vi "UHR-Fleezers Control (host) -TL - oscillation.vi"(0 "Tab Control":T5(tab)) -> ()   [LabVIEW 2013] (continued)
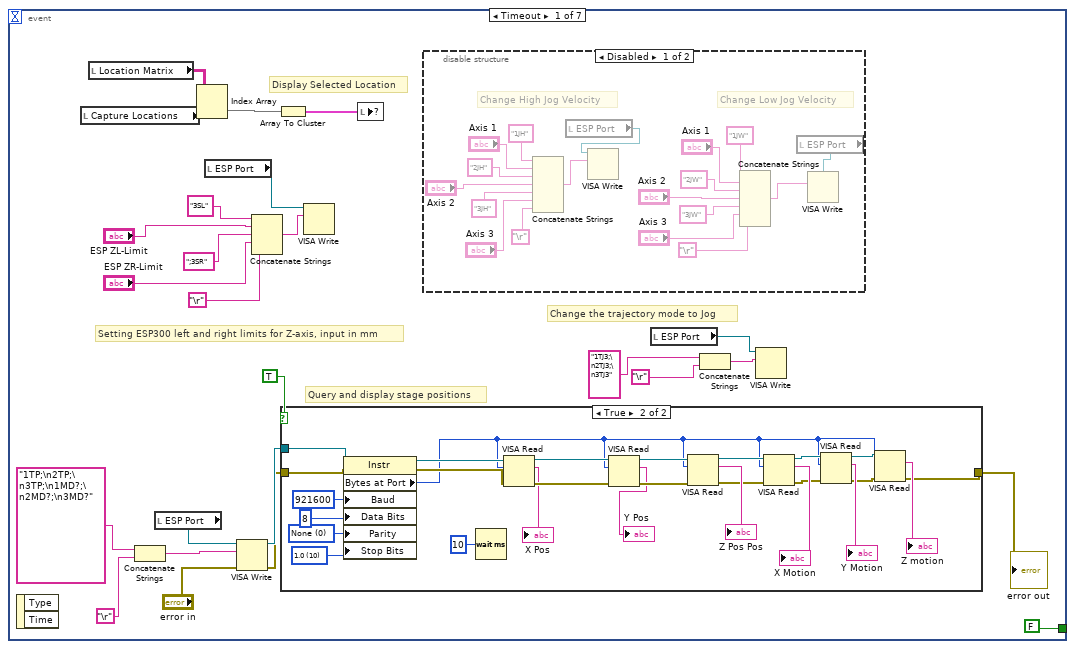
[diagram p3: hidden frame]
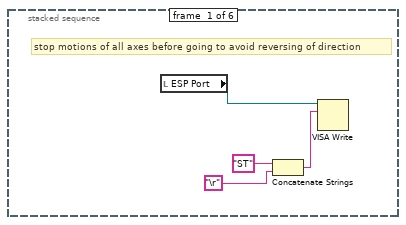
[diagram p6: hidden frame]
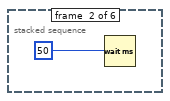
[diagram p7: hidden frame]
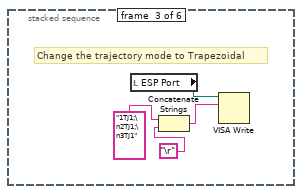
[diagram p8: hidden frame]
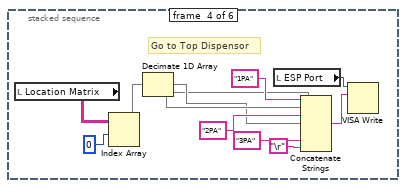
[diagram p9: hidden frame]
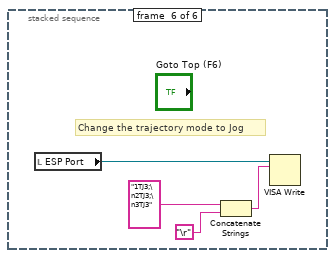
[diagram p10: hidden frame]
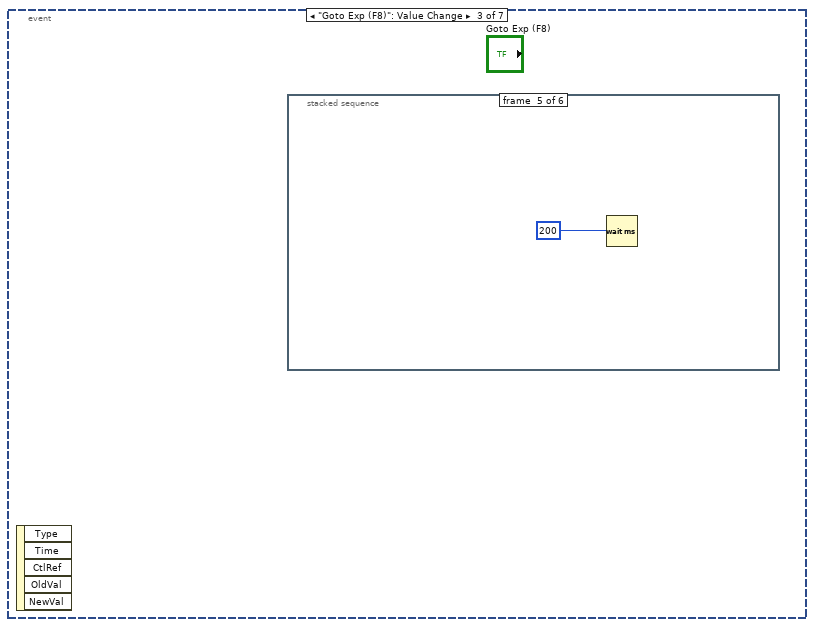
[diagram p11: hidden frame]
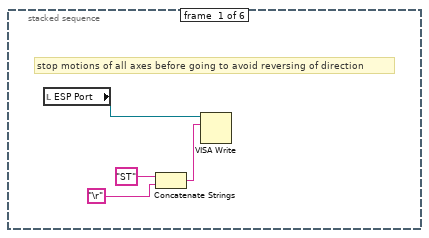
[diagram p12: hidden frame]
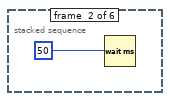
[diagram p13: hidden frame]
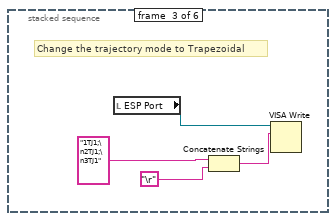
[diagram p14: hidden frame]
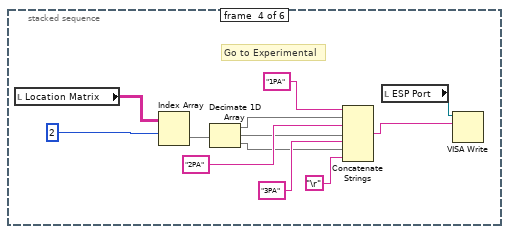
[diagram p15: hidden frame]
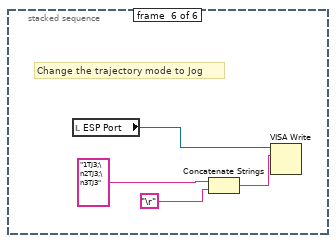
[diagram p16: hidden frame]
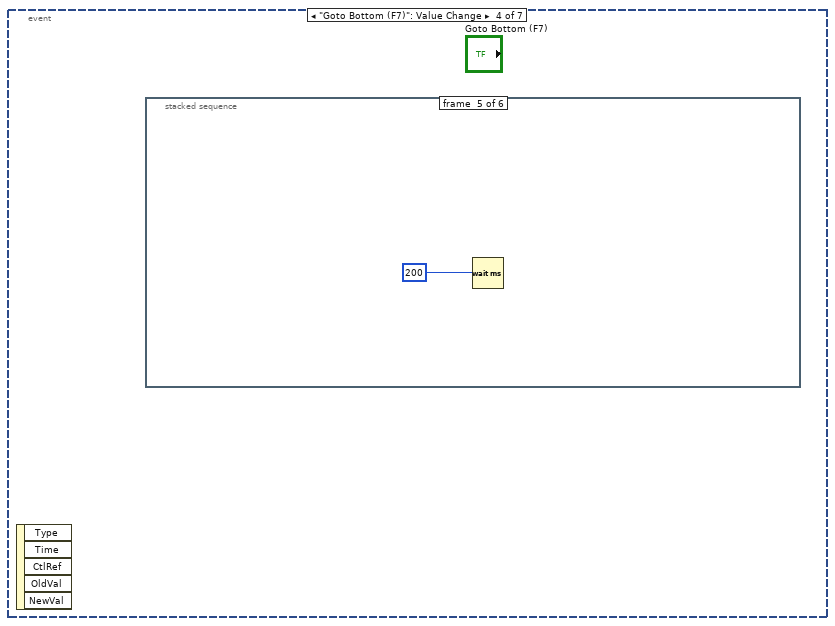
[diagram p17: hidden frame]
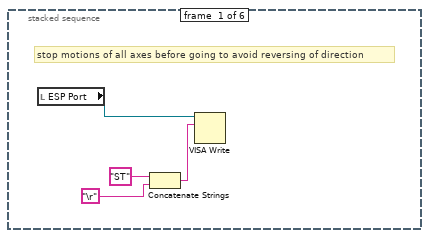
[diagram p18: hidden frame]
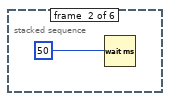
[diagram p19: hidden frame]
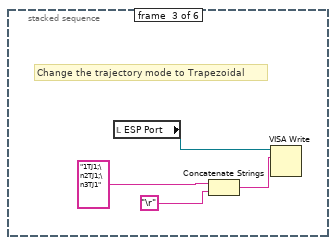
[diagram p20: hidden frame]
            n1984 = local write "Save index"(w3239) -> ()
            n1985 = Array Size(array=w3250) -> (size(s)=w3251:i32)
            n1986 = Open/Create/Replace File(file path (use dialog)=w3226, operation (0:open)=T23."create", access (0:read/write)=enum16{"read/write", "read-only", "write-only"}."write-only") -> (refnum out=w3264:refnum<file>)  [unwired: 1 in, 4 out]
            n1987 = local write "Saving..."(TRUE ("Saving...")) -> ()
            n1988 = To Double Precision Float(number=w3251) -> (double precision float=w3249:dbl)
            n1989 = String Length(string="Comment (data description)") -> (length=w3247:i32)
            n1990 = To Double Precision Float(number=w3247) -> (double precision float=w3246:dbl)
            n1991 = Deny Access(7:w3264) -> (3:w3263:refnum<file>)  [unwired: 1 in, 2 out]
            n1992 = Build Array (concatenate)(w3249, w3250, w3246) -> (w3248:dbl[])
            n1993 = case "If fluorescence data to be saved" shown="True" w3237 {
              tunnel: w3226 -> [_ w3316]
              tunnel: [refnum<k0> refnum w3296] -> w3238
              frame False {
              }
              frame True {
                w3295 = 0.0
                n1994 = local read "APD Integration Time (s)"() -> (w3301:dbl)
                n1995 = local read "N APD Samp/step"() -> (w3294:dbl)
                n1996 = Path To String(path=w3316) -> (string=w3315:string)
                n1997 = String Length(string=w3315) -> (length=w3314:i32)
                n1998 = Subtract(x=w3314, y=4) -> (x-y=w3312:i32)
                n1999 = String Subset(string=w3315, length (rest)=w3312) -> (substring=w3311:string)  [unwired: 1 out]
                n2000 = Build Array(w3301, w3294, w3295, w3295, w3295, w3295, w3295, w3295) -> (w3298:dbl[])
                n2001 = Concatenate Strings(w3311, "_fl.dat" ("string")) -> (w3309:string)
                n2002 = Array Size(array=w3298) -> (size(s)=w3300:i32)
                n2003 = String To Path(string=w3309) -> (path=w3305:path)
                n2004 = Open/Create/Replace File(file path (use dialog)=w3305, operation (0:open)=T23."create", access (0:read/write)=enum16{"read/write", "read-only", "write-only"}."write-only") -> (refnum out=w3306:refnum<file>)  [unwired: 1 in, 4 out]
                n2005 = Deny Access(7:w3306) -> (3:w3302:refnum<file>)  [unwired: 1 in, 2 out]
                n2006 = To Double Precision Float(number=w3300) -> (double precision float=w3299:dbl)
                n2007 = Build Array (concatenate)(w3299, w3298) -> (w3297:dbl[])
                n2008 = Write to Binary File(file (use dialog)=w3302, data=w3297, 5:FALSE ("prepend array or string size? (T)"), 9:T29."big-endian, network order" ("byte order (0:big-endian, network order)")) -> (refnum out=w3296:refnum<file>)  [unwired: 1 in, 3 out]
              }
            }
            n2009 = case shown="True" w3224 {
              tunnel: w3226 -> [_ w3278]
              tunnel: [refnum<k0> refnum w3277] -> w3225
              frame False {
              }
              frame True {
                w3273 = 0.0 ("element")
                n2010 = Path To String(path=w3278) -> (string=w3292:string)
                n2011 = Build Array(w3273, w3273, w3273, w3273, w3273, w3273, w3273, w3273) -> (w3274:dbl[])
                n2012 = String Length(string=w3292) -> (length=w3291:i32)
                n2013 = Subtract(x=w3291, y=4) -> (x-y=w3289:i32)
                n2014 = Array Size(array=w3274) -> (size(s)=w3276:i32)
                n2015 = String Subset(string=w3292, length (rest)=w3289) -> (substring=w3288:string)  [unwired: 1 out]
                n2016 = To Double Precision Float(number=w3276) -> (double precision float=w3275:dbl)
                n2017 = Concatenate Strings(w3288, "_pos.dat" ("string")) -> (w3286:string)
                n2018 = Build Array (concatenate)(w3275, w3274) -> (w3272:dbl[])
                n2019 = String To Path(string=w3286) -> (path=w3282:path)
                n2020 = Open/Create/Replace File(file path (use dialog)=w3282, operation (0:open)=T23."create", access (0:read/write)=enum16{"read/write", "read-only", "write-only"}."write-only") -> (refnum out=w3283:refnum<file>)  [unwired: 1 in, 4 out]
                n2021 = Deny Access(7:w3283) -> (3:w3279:refnum<file>)  [unwired: 1 in, 2 out]
                n2022 = Write to Binary File(file (use dialog)=w3279, data=w3272, 5:FALSE ("prepend array or string size? (T)"), 9:T29."big-endian, network order" ("byte order (0:big-endian, network order)")) -> (refnum out=w3277:refnum<file>)  [unwired: 1 in, 3 out]
              }
            }
            n2023 = Write to Binary File(file (use dialog)=w3263, data=w3248, 5:w3244, 9:w3242) -> (refnum out=w3245:refnum<file>)  [unwired: 1 in, 3 out]
            n2024 = Write to Binary File(file (use dialog)=w3245, data="Comment (data description)", 5:w3244, 9:w3242) -> (refnum out=w3241:refnum<file>)  [unwired: 1 in, 3 out]
          }
        }
        n2025 = feedback-in #19(w3184) -> ()
        n2026 = feedback-in #20(w3211) -> ()
        n2027 = feedback-in #21(w3183) -> ()
        n2028 = feedback-in #22(w3194) -> ()
        n2029 = feedback-in #23(w3197) -> ()
        n2030 = feedback-in #24(w3210) -> ()
        n2031 = feedback-in #25(w3200) -> ()
      }
      frame #1 {
        n2032 = local read "Saving..."() -> (w3441:bool)
        n2033 = case shown="True" w3441 {
          tunnel: w3445 -> [_ w3455]
          tunnel: w3444 -> [_ w3469]
          tunnel: w3443 -> [_ w3465]
          tunnel: w3442 -> [_ w3464]
          tunnel: w3440 -> [_ w3463]
          tunnel: w3439 -> [_ w3458]
          tunnel: w3438 -> [_ w3457]
          tunnel: w3437 -> [_ w3456]
          tunnel: w3436 -> [_ w3454]
          tunnel: w3435 -> [_ w3452]
          tunnel: w3434 -> [_ w3451]
          tunnel: w3433 -> [_ w3450]
          tunnel: w3432 -> [_ w3449]
          tunnel: w3431 -> [_ w3448]
          tunnel: w3430 -> [_ w3447]
          tunnel: w3429 -> [_ w3446]
          frame False {
          }
          frame True {
            n2034 = Multiply(x=w3455, y=w3454) -> (x*y=→"Time (s)":dbl)
            n2035 = Less Or Equal?(x=w3455, y=w3463) -> (x <= y?=w3467:bool)
            n2036 = Or(x="Stop Saving", y="Abort save 2") -> (x .or. y?=w3459:bool)
            n2037 = Not(x=w3459) -> (.not. x?=w3468:bool)
            n2038 = And(x=w3467, y=w3468) -> (x .and. y?=w3466:bool)
            n2039 = case shown="True" w3466 {
              tunnel: w3469 -> [w3476 w3544]
              tunnel: [0.0 w3547] -> w3462
              tunnel: w3455 -> [_ w3545]
              tunnel: w3463 -> [_ w3546]
              tunnel: w3465 -> [_ w3541]
              tunnel: w3464 -> [_ _]
              tunnel: w3458 -> [w3474 w3534]
              tunnel: w3457 -> [w3473 w3535]
              tunnel: w3456 -> [_ w3533]
              tunnel: w3452 -> [_ w3532]
              tunnel: w3451 -> [_ w3486]
              tunnel: w3450 -> [_ w3525]
              tunnel: w3449 -> [_ w3503]
              tunnel: w3448 -> [w3471 w3484]
              tunnel: w3447 -> [w3472 w3483]
              tunnel: w3446 -> [_ w3480]
              frame False {
                w3470 = FALSE
                n2040 = Close File(refnum=w3476) -> ()  [unwired: 1 in, 2 out]
                n2041 = case shown="True" w3473 {
                  tunnel: w3474 -> [_ w3478]
                  frame False {
                  }
                  frame True {
                    n2042 = Close File(refnum=w3478) -> ()  [unwired: 1 in, 2 out]
                  }
                }
                n2043 = case shown="True" w3471 {
                  tunnel: w3472 -> [_ w3477]
                  frame False {
                  }
                  frame True {
                    n2044 = Close File(refnum=w3477) -> ()  [unwired: 1 in, 2 out]
                  }
                }
                n2045 = local write "Calibrating Trap..."(w3470) -> ()
                n2046 = call <vilib>:"Beep.vi"() -> ()  [unwired: 3 in, 9 out]
                n2047 = local write "Stop Saving"(w3470) -> ()
                n2048 = property on="Raster Scanning..." class="Bool (strict)"("Val(Sgnl)"=w3470) -> ()  [unwired: 2 in, 2 out]
                "Saving..." <- w3470
              }
              frame True {
                n2049 = local read "Calibrating Trap..."() -> (w3536:bool)
                n2050 = case "Write fl. data" shown="True" w3535 {
                  tunnel: w3534 -> [_ w3570]
                  tunnel: w3533 -> [_ w3569]
                  frame False {
                  }
                  frame True {
                    n2051 = Write to Binary File(file (use dialog)=w3570, data=w3569, 5:FALSE ("prepend array or string size? (T)"), 9:T29."big-endian, network order" ("byte order (0:big-endian, network order)")) -> ()  [unwired: 1 in, 4 out]
                  }
                }
                n2052 = Greater?(x="Save ave N", y=1.0) -> (0:w3539:bool)
                n2053 = Not(x=w3536) -> (.not. x?=w3538:bool)
                n2054 = And(x=w3538, y=w3539) -> (x .and. y?=w3481:bool)
                n2055 = case shown="True" w3481 {
                  tunnel: w3480 -> [w3550 w3561]
                  tunnel: [w3550 w3553] -> w3479
                  tunnel: "Save ave N" -> [_ w3554]
                  frame False {
                  }
                  frame True {
                    w3551 = 2 ("dimension size")
                    n2056 = Array Size(array=w3561) -> (size(s)=w3555:i32)
                    n2057 = Divide(x=w3555, y=w3551) -> (x/y=w3559:dbl)
                    n2058 = Reshape Array(w3561, w3559, w3551) -> (w3560:u64[][])
                    n2059 = Transpose 2D Array(2D array=w3560) -> (transposed array=w3558:u64[][])
                    n2060 = for {
                      tunnel: w3558 -> [w3563] mode=indexing
                      tunnel: [w3562] -> w3552 mode=indexing
                      tunnel: w3554 -> [w3564]
                      workers-P: _ -> [_]
                      n2061 = call "downsample 1D array - U64.vi"("Ave N"=w3564, "Array In"=w3563) -> ("Array Out"=w3562:u64[])  [unwired: 1 in]
                    }
                    n2062 = Transpose 2D Array(2D array=w3552) -> (transposed array=w3557:u64[][])
                    n2063 = Divide(x=w3555, y=w3554) -> (x/y=w3556:dbl)
                    n2064 = Reshape Array(w3557, w3556) -> (w3553:u64[])
                  }
                }
                n2065 = case shown="False" w3481 {
                  tunnel: w3541 -> [w3573 w3585]
                  tunnel: [w3573 w3577] -> w3537
                  tunnel: "Save ave N" -> [_ w3578]
                  tunnel: w3532 -> [_ w3576]
                  frame False {
                    # "don't downsample data for trap calibration"
                  }
                  frame True {
                    n2066 = Array Size(array=w3585) -> (size(s)=w3579:i32)
                    n2067 = Array Size(array=w3576) -> (size(s)=w3575:i32)
                    n2068 = Divide(x=w3579, y=w3575) -> (x/y=w3583:dbl)
                    n2069 = Reshape Array(w3585, w3583, w3575) -> (w3584:i16[][])
                    n2070 = Transpose 2D Array(2D array=w3584) -> (transposed array=w3582:i16[][])
                    n2071 = for {
                      tunnel: w3582 -> [w3588] mode=indexing
                      tunnel: [w3587] -> w3574 mode=indexing
                      tunnel: w3578 -> [w3586]
                      workers-P: _ -> [_]
                      n2072 = call "downsample 1D array - I16.vi"("Ave N"=w3586, "Array In"=w3588) -> ("Array Out"=w3587:i16[])  [unwired: 1 out]
                    }
                    n2073 = Transpose 2D Array(2D array=w3574) -> (transposed array=w3581:i16[][])
                    n2074 = Divide(x=w3579, y=w3578) -> (x/y=w3580:dbl)
                    n2075 = Reshape Array(w3581, w3580) -> (w3577:i16[])
                  }
                }
                n2076 = Index Array(array=w3503, index=1) -> (element=w3506:waveform(dbl))
                n2077 = Index Array(array=w3503, index=0) -> (element=w3508:waveform(dbl))
                n2078 = Unbundle By Name(w3506) -> ("Y"=w3510:dbl[])
                n2079 = Unbundle By Name(w3508) -> ("Y"=w3518:dbl[])
                n2080 = case "Write trap pos. data" shown="True" w3484 {
                  tunnel: w3483 -> [_ w3566]
                  tunnel: w3479 -> [_ w3565]
                  frame False {
                  }
                  frame True {
                    n2081 = Write to Binary File(file (use dialog)=w3566, data=w3565, 5:FALSE ("prepend array or string size? (T)"), 9:T29."big-endian, network order" ("byte order (0:big-endian, network order)")) -> ()  [unwired: 1 in, 4 out]
                  }
                }
                n2082 = Write to Binary File(file (use dialog)=w3544, data=w3537, 5:FALSE ("prepend array or string size? (T)"), 9:T29."big-endian, network order" ("byte order (0:big-endian, network order)")) -> ()  [unwired: 1 in, 4 out]
                n2083 = feedback #26(w3510) -> (w3512:dbl[])
                n2084 = Build Array (concatenate)(w3512, w3510) -> (w3511:dbl[])
                n2085 = Select(t=w3510, s=w3486, f=w3511) -> (s? t:f=w3496:dbl[])
                n2086 = feedback-in #26(w3496) -> ()
                n2087 = feedback #27(w3518) -> (w3531:dbl[])
                n2088 = Build Array (concatenate)(w3531, w3518) -> (w3530:dbl[])
                n2089 = Select(t=w3518, s=w3486, f=w3530) -> (s? t:f=w3505:dbl[])
                n2090 = feedback-in #27(w3505) -> ()
                n2091 = Divide(x=w3545, y=w3546) -> (x/y=w3548:dbl)
                n2092 = Multiply(x=w3548, y=100.0) -> (x*y=w3547:dbl)
                n2093 = Build Array(w3505, w3496) -> (→"Saved APD":dbl[][])
                n2094 = Array Size(array=w3505) -> (size(s)=w3523:i32)
                n2095 = Unbundle By Name(w3525) -> ("Y"=w3529:dbl[])
                n2096 = Subtract(x=w3523, y="N pts to average") -> (x-y=w3499:i32)
                n2097 = Multiply(x="N pts to average", y=u16 2) -> (x*y=w3500:u16)
                n2098 = Subtract(x=w3523, y=w3500) -> (x-y=w3498:i32)
                n2099 = feedback #28(w3529) -> (w3528:dbl[])
                n2100 = Build Array (concatenate)(w3528, w3529) -> (w3527:dbl[])
                n2101 = Select(t=w3529, s=w3486, f=w3527) -> (s? t:f=w3526:dbl[])
                "Trap Delta Graph" <- w3526
                n2102 = feedback-in #28(w3526) -> ()
                n2103 = Array Subset(array=w3505, index=w3499, length="N pts to average") -> (w3522:dbl[])
                n2104 = Array Subset(array=w3505, index=w3498, length="N pts to average") -> (w3521:dbl[])
                n2105 = Array Subset(array=w3496, index=w3499, length="N pts to average") -> (w3502:dbl[])
                n2106 = Array Subset(array=w3496, index=w3498, length="N pts to average") -> (w3501:dbl[])
                n2107 = call-poly <vilib>:"Mean.vi"("X"=w3522) -> ("mean"=w3520:dbl)  [unwired: 1 out]
                n2108 = call-poly <vilib>:"Mean.vi"("X"=w3502) -> ("mean"=w3495:dbl)  [unwired: 1 out]
                n2109 = call-poly <vilib>:"Mean.vi"("X"=w3521) -> ("mean"=w3519:dbl)  [unwired: 1 out]
                n2110 = call-poly <vilib>:"Mean.vi"("X"=w3501) -> ("mean"=w3494:dbl)  [unwired: 1 out]
                n2111 = Subtract(x=w3495, y=w3494) -> (x-y=w3485:dbl)
                "Delta Fl. 2" <- w3485
                n2112 = Subtract(x=w3520, y=w3519) -> (x-y=w3517:dbl)
                "Delta Fl. 1" <- w3517
                n2113 = Initialize Array(w3517, 1 ("dimension size")) -> (w3514:dbl[])
                n2114 = Initialize Array(w3485, 1 ("dimension size")) -> (w3491:dbl[])
                n2115 = feedback #29(w3514) -> (w3515:dbl[])
                n2116 = Build Array (concatenate)(w3515, w3514) -> (w3513:dbl[])
                n2117 = feedback #30(w3491) -> (w3492:dbl[])
                n2118 = Build Array (concatenate)(w3492, w3491) -> (w3490:dbl[])
                n2119 = Select(t=w3514, s=w3486, f=w3513) -> (s? t:f=w3489:dbl[])
                n2120 = feedback-in #29(w3489) -> ()
                n2121 = Select(t=w3491, s=w3486, f=w3490) -> (s? t:f=w3488:dbl[])
                n2122 = feedback-in #30(w3488) -> ()
                n2123 = Build Array(w3489, w3488) -> (→"Save APD Deriv":dbl[][])
              }
            }
            "Progress" <- w3462
            "Progress 2" <- w3462
          }
        }
      }
    }
    n2124 = Bundle By Name(cluster=w2208, "Green FB Ch 0"=w2207, "Green FB Ch 1"=w2206) -> (w2186:T48)
    "Green FB Signals (V)" <- w2186
    n2125 = Unbundle By Name(w2186) -> ("Green FB Ch 2"=→"Green FB Plot":dbl)
    n2126 = local read "wait to reset values"() -> (w2276:bool)
    n2127 = Not(x=w2273) -> (.not. x?=w2277:bool)
    n2128 = And(x=w2277, y=w2276) -> (x .and. y?=w2278:bool)
    n2129 = case "Part of MCL raster scanning: returns to initial positions after scan done" shown="False" w2278 {
      tunnel: w2281 -> [w3014 w3021]
      tunnel: [w3014 w3020] -> w2280
      tunnel: w2275 -> [w3013 w3019]
      tunnel: [w3013 w3018] -> w2274
      frame False {
      }
      frame True {
        w3029 = 10.0 ("y")
        w3028 = 32767.0 ("y")
        # "to return scan values\nafter a synchronous \nAOM scan"
        n2130 = local read "AO2"() -> (w3022:dbl)
        n2131 = local read "AO1"() -> (w3023:dbl)
        n2132 = local write "wait to reset values"(FALSE ("wait to reset values")) -> ()
        n2133 = Multiply(x=w3023, y=w3028) -> (x*y=w3025:dbl)
        n2134 = Multiply(x=w3022, y=w3028) -> (x*y=w3027:dbl)
        n2135 = Divide(x=w3025, y=w3029) -> (x/y=w3024:dbl)
        n2136 = Divide(x=w3027, y=w3029) -> (x/y=w3026:dbl)
        n2137 = To Word Integer(number=w3024) -> (16bit integer=w3030:i16)
        n2138 = To Word Integer(number=w3026) -> (16bit integer=w3031:i16)
        n2139 = local read "Total Counts (ticks)"() -> (w3015:u32)
        n2140 = xnode "Read/Write Control"("FPGA VI Reference In"=w3021, "error in"=w3019, "AO1"=w3030, "AO2"=w3031, "MCL count"=w3015) -> ("FPGA VI Reference Out"=w3020:T19, "error out"=w3018:errorcluster)
        n2141 = local read "Scan Range (V)\n(of steps)"() -> (w3016:dbl)
        n2142 = property on="Scan Range (V)\n(of steps)" class="DigNum (strict)"("Val(Sgnl)"=w3016) -> ()  [unwired: 2 in, 2 out]
      }
    }
    n2143 = node-c288() -> ()  [unwired: 2 out]
  }
  n2144 = node-c288(3 ("Processor")) -> (w77:T24)  [unwired: 3 out]
  n2145 = timed-loop "Oscillate AOD (debugging)" {
    tunnel: w2 -> [w3590]
    tunnel: [w3589] -> w40
    timing: w77 -> [_]
    timing-out: [_] -> w76
    stop <- w3589 stop-if-true
    n2146 = node-c288() -> ()  [unwired: 2 out]
    n2147 = event shown="[0] \"Oscillate Traps\", \"Fish for Tether\": Value Change" {
      selector: _ -> [_ _ _]
      dyn-events: _ -> [_ _ _]
      timeout: _ -> [_ _ _]
      tunnel: w3590 -> [w3597 _ _]
      tunnel: [FALSE ("Stop All") _ w3869] -> w3589
      event "Oscillate Traps", "Fish for Tether": Value Change {
        n2148 = event-data() -> ()  [unwired: 6 out]
        n2149 = local read "Oscillate Traps"() -> (w3596:bool)
        n2150 = Or(x=w3596, y="Fish for Tether") -> (x .or. y?=w3594:bool)
        n2151 = case shown="True" w3594 {
          tunnel: w3597 -> [_ w3600]
          tunnel: "Fish for Tether" -> [_ w3599]
          frame False {
          }
          frame True {
            n2152 = case shown="True" w3599 {
              frame False {
              }
              frame True {
                n2153 = local write "Scan axis (osc)"(TRUE) -> ()
                n2154 = local write "Tether"(FALSE ("Tether")) -> ()
              }
            }
            n2155 = node-c288("Time Step (ms)") -> (w3602:T24)  [unwired: 3 out]
            n2156 = timed-loop "Oscillate AOD" {
              timing: w3602 -> [_]
              timing-out: [_] -> w3601
              tunnel: w3600 -> [w3612]
              tunnel: w3599 -> [w3611]
              i -> [w3614]
              stop <- w3610 stop-if-true
              n2157 = node-c288() -> (w3613:i64)  [unwired: 1 out]
              n2158 = flat-sequence {
                tunnel: w3614 -> [w3643]
                tunnel: w3613 -> [w3642]
                tunnel: w3612 -> [w3628]
                tunnel: w3611 -> [w3630]
                tunnel: [w3630] -> w3609
                tunnel: [w3629] -> w3608
                tunnel: [w3627] -> w3607
                tunnel: [w3624] -> w3605
                tunnel: w3609 -> [w3680]
                tunnel: w3608 -> [w3678]
                tunnel: w3607 -> [w3677]
                tunnel: [w3676] -> w3606
                tunnel: w3605 -> [w3675]
                tunnel: [w3744] -> w3610
                tunnel: w3606 -> [w3742]
                frame #0 {
                  # "Also note that the 1 ms lower limit per iteration of all LabView loops\nis the reason why the power spectrum shows higher harmonics\nwhen performing a forced oscillation-based calibration procedure.\nOne solution to this would be to implement the osciallation using\nthe FPGA, or to account for the harmonics in the analysis. The forced\noscillation needs to discretized on timescales that won't affect\nthe power spectrum (i.e., > 66 kHz detection bandwidth; < 15 µs)."
                  # "Note: Trap Oscillation was originally written\nfor Trap 2!!!  This was modified to oscillation\nboth traps for board 1 (x-axis), but not changed\nfor board 2 (y-axis), since we only implement\nx-axis control at the moment (TL, 1/1/15)"
                  n2159 = Divide(x=w3642, y=i64 1000) -> (x/y=w3637:dbl)
                  n2160 = Multiply(x=w3637, y=w3643) -> (x*y=w3639:dbl)
                  n2161 = Multiply(x="Osc. freq. (Hz)", y=6.283185307179586) -> (x*y=w3640:dbl)
                  n2162 = Multiply(x=w3640, y=w3639) -> (x*y=w3626:dbl)
                  n2163 = local read "BD 1 Frequency 1 (MHz)"() -> (w3616:dbl)
                  n2164 = local read "BD 1 Frequency 2 (MHz)"() -> (w3623:dbl)
                  n2165 = case shown="False" w3630 {
                    tunnel: w3626 -> [w3649 w3657]
                    tunnel: w3623 -> [_ w3667]
                    tunnel: [w3644 w3651] -> w3618
                    tunnel: [FALSE w3660] -> w3627
                    tunnel: [0.0 w3653] -> w3624
                    tunnel: w3616 -> [_ w3652]
                    tunnel: [w3644 0.0 ("y")] -> w3615
                    frame False {
                      n2166 = Sine(x=w3649) -> (sin(x)=w3647:dbl)
                      n2167 = Multiply(x=w3647, y="Osc. amp. (MHz)") -> (x*y=w3644:dbl)
                    }
                    frame True {
                      n2168 = Cosine(x=w3657) -> (cos(x)=w3670:dbl)
                      n2169 = Subtract(x=w3667, y=w3652) -> (x-y=w3666:dbl)
                      n2170 = Decrement(x=w3670) -> (x-1=w3669:dbl)
                      n2171 = Subtract(x=w3666, y="Closest Delta (MHz)") -> (x-y=w3663:dbl)
                      n2172 = Divide(x=w3669, y=2.0) -> (x/y=w3664:dbl)
                      n2173 = Multiply(x=w3664, y=w3663) -> (x*y=w3651:dbl)
                      n2174 = local read "Vec Mean of T1 T2"() -> (w3659:dbl[])
                      n2175 = Greater?(x=w3659, y="Stop F (pN)") -> (0:w3661:bool[])
                      n2176 = Or Array Elements(Boolean array=w3661) -> (logical OR=w3660:bool)
                      n2177 = Divide(x=w3657, y=6.283185307179586) -> (x/y=w3656:dbl)
                      n2178 = Round Toward +Infinity(x=w3656) -> (ceil(x): smallest int >= x=w3653:dbl)
                      "Attempts" <- w3653
                      n2179 = Greater?(x=w3653, y="Attempt Limit") -> (0:w3655:bool)
                      n2180 = case shown="True" w3655 {
                        frame False {
                        }
                        frame True {
                          n2181 = local write "Fish for Tether"(FALSE ("Fish for Tether")) -> ()
                          n2182 = call <vilib>:"Beep.vi"() -> ()  [unwired: 3 in, 9 out]
                          n2183 = local read "Messages"() -> (w3672:string)
                          n2184 = call "Update messages.vi"("Message to add"="Tether fishing timeout." ("Messages"), "Old message string"=w3672) -> ("New message string"=→"Messages":string)
                        }
                      }
                    }
                  }
                  n2185 = Add(x=w3615, y=w3616) -> (x+y=w3620:dbl)
                  n2186 = Select(t=w3620, s="Scan axis (osc)", f=w3616) -> (s? t:f=w3617:dbl)
                  n2187 = local read "Y RF Frequency Limits (MHz)"() -> (w3631:T16)
                  n2188 = local read "X RF Frequency Limits (MHz)"() -> (w3632:T16)
                  n2189 = local read "BD 2 Frequency 2 (MHz)"() -> (w3622:dbl)
                  n2190 = Select(t=w3623, s="Scan axis (osc)", f=w3622) -> (s? t:f=w3633:dbl)
                  n2191 = Add(x=w3618, y=w3633) -> (x+y=w3629:dbl)
                  n2192 = Select(t=w3629, s="Scan axis (osc)", f=w3623) -> (s? t:f=w3621:dbl)
                  n2193 = Select(t=w3622, s="Scan axis (osc)", f=w3629) -> (s? t:f=w3634:dbl)
                  n2194 = local read "BD 2 Frequency 3 (MHz)"() -> (w3635:dbl)
                  n2195 = local read "BD 1 Frequency 3 (MHz)"() -> (w3636:dbl)
                  n2196 = call "set RF board frequency - interlace.vi"("Board 2 Frequency Limits"=w3631, "Board 1 Frequency Limits"=w3632, "FPGA VI Reference In"=w3628, "Board 2 Frequency 3 (MHz)"=w3635, "Board 1 Frequency 3 (MHz)"=w3636, "Board 2 Frequency 2 (MHz)"=w3622, "Board 2 Frequency 1 (MHz)"=w3634, "Board 1 Frequency 2 (MHz)"=w3621, "Board 1 Frequency 1  (MHz)"=w3617) -> ()  [unwired: 1 in, 2 out]
                }
                frame #1 {
                  n2197 = And(x=w3680, y=w3677) -> (x .and. y?=w3679:bool)
                  n2198 = case "Only if were fishing and now formed tether" shown="True" w3679 {
                    tunnel: w3678 -> [w3682 w3694]
                    tunnel: [w3681 w3693] -> w3676
                    tunnel: w3675 -> [_ w3689]
                    frame False {
                      n2199 = local read "Fish for Tether"() -> (w3681:bool)
                      n2200 = case shown="True" w3681 {
                        tunnel: w3682 -> [_ _]
                        frame False {
                        }
                        frame True {
                        }
                      }
                    }
                    frame True {
                      w3693 = FALSE ("Fish for Tether")
                      n2201 = call <vilib>:"Beep.vi"() -> ()  [unwired: 3 in, 9 out]
                      n2202 = Number To Decimal String(number=w3689, width (-)=i16 1) -> (decimal integer string=w3687:string)
                      n2203 = case shown="\"2\", \"3\", \"4\", \"5\", \"6\"" "Then..." {
                        selector: "Then..." -> [_ w3697]
                        tunnel: w3694 -> [w3696 _]
                        frame "1", Default {
                          # "do nothing"
                          n2204 = property on="BD 1 Frequency 1 (MHz)" class="DigNum (strict)"("Val(Sgnl)"=w3696) -> ()  [unwired: 2 in, 2 out]
                        }
                        frame "2", "3", "4", "5", "6" {
                          n2205 = flat-sequence {
                            tunnel: w3697 -> [w3699]
                            frame #0 {
                              n2206 = property on="Trap Delta (MHz)" class="DigNum (strict)"("Val(Sgnl)"="Move to Delta 1 (MHz)") -> ()  [unwired: 2 in, 2 out]
                            }
                            frame #1 {
                              n2207 = case shown="\"5\", \"6\"" w3699 {
                                selector: w3699 -> [w3702 w3712 _]
                                frame "3", "4" {
                                n2208 = flat-sequence {
                                tunnel: w3702 -> [w3703]
                                tunnel: [w3703] -> w3700
                                tunnel: [w3705] -> w3701
                                tunnel: w3700 -> [w3705]
                                tunnel: w3701 -> [w3709]
                                frame #0 {
                                n2209 = property on="Green Laser ON/Interlacing" class="Bool (strict)"("Val(Sgnl)"=TRUE ("Value (Signaling)")) -> ()  [unwired: 2 in, 2 out]
                                }
                                frame #1 {
                                n2210 = Multiply(x="Wait Before Save (s)", y=u32 1000 ("x")) -> (x*y=w3707:u32)
                                n2211 = Wait (ms)(milliseconds to wait=w3707) -> ()  [unwired: 1 out]
                                }
                                frame #2 {
                                n2212 = property on="Start Saving" class="Bool (strict)"("Value"=TRUE ("Start Saving")) -> ()  [unwired: 2 in, 2 out]
                                n2213 = case shown="Default" w3709 {
                                frame Default {
                                }
                                frame "4" {
                                n2214 = property on="Fl. Triggered..." class="Bool (strict)"("Val(Sgnl)"=TRUE ("Value (Signaling)")) -> ()  [unwired: 2 in, 2 out]
                                }
                                }
                                }
                                }
                                }
                                frame "5", "6" {
                                n2215 = stacked-sequence {
                                tunnel: w3712 -> [_ _ _ _ _ _ _ _ w3729 _ _]
                                frame #0 {
                                n2216 = Replace Array Subset(array=u32[] [0] ("Index Values"), new element="Raster Set Upon Tether", index=0) -> (w3713:u32[])
                                n2217 = property on="Saved AOD Raster Scan Parameter Sets" class="Arr (strict)"("Index Values"=w3713) -> ()  [unwired: 2 in, 2 out]
                                }
                                frame #1 {
                                n2218 = Wait (ms)(milliseconds to wait=u32 500) -> ()  [unwired: 1 out]
                                }
                                frame #2 {
                                n2219 = property on="Load parameters" class="Bool (strict)"("Val(Sgnl)"=TRUE ("Value (Signaling)")) -> ()  [unwired: 2 in, 2 out]
                                }
                                frame #3 {
                                n2220 = Wait (ms)(milliseconds to wait=u32 500) -> ()  [unwired: 1 out]
                                }
                                frame #4 {
                                n2221 = property on="Trap Raster Scan" class="Bool (strict)"("Val(Sgnl)"=TRUE ("Value (Signaling)")) -> ()  [unwired: 2 in, 2 out]
                                }
                                frame #5 {
                                n2222 = Wait (ms)(milliseconds to wait=u32 2000) -> ()  [unwired: 1 out]
                                }
                                frame #6 {
                                n2223 = while {
                                stop <- w3724 stop-if-true
                                n2224 = local read "Raster Scanning..."() -> (w3723:bool)
                                n2225 = local read "Saving..."() -> (w3726:bool)
                                n2226 = Wait (ms)(milliseconds to wait=u32 100) -> ()  [unwired: 1 out]
                                n2227 = Not(x=w3726) -> (.not. x?=w3725:bool)
                                n2228 = Not(x=w3723) -> (.not. x?=w3722:bool)
                                n2229 = And(x=w3725, y=w3722) -> (x .and. y?=w3724:bool)
                                }
                                }
                                frame #7 {
                                n2230 = property on="Trap Delta (MHz)" class="DigNum (strict)"("Val(Sgnl)"="Move to Delta 2 (MHz)") -> ()  [unwired: 2 in, 2 out]
                                }
                                frame #8 {
                                n2231 = local read "Tether"() -> (w3730:bool)
                                n2232 = case shown="True" w3730 {
                                tunnel: w3729 -> [_ w3731]
                                frame False {
                                }
                                frame True {
                                n2233 = flat-sequence {
                                tunnel: w3731 -> [w3733]
                                frame #0 {
                                n2234 = Wait (ms)(milliseconds to wait=u32 500) -> ()  [unwired: 1 out]
                                }
                                frame #1 {
                                n2235 = case shown="\"6\"" w3733 {
                                frame Default {
                                }
                                frame "6" {
                                n2236 = property on="Green Laser ON/Interlacing" class="Bool (strict)"("Val(Sgnl)"=TRUE ("Green Laser ON/Interlacing")) -> ()  [unwired: 2 in, 2 out]
                                }
                                }
                                }
                                frame #2 {
                                n2237 = Wait (ms)(milliseconds to wait=u32 500) -> ()  [unwired: 1 out]
                                }
                                frame #3 {
                                n2238 = local write "Start Saving"("Save at end (5, 6)") -> ()
                                }
                                }
                                }
                                }
                                }
                                frame #9 {
                                n2239 = local read "Bead Sep. Int. Time (s)"() -> (w3739:dbl)
                                n2240 = Multiply(x=w3739, y=1000.0) -> (x*y=w3738:dbl)
                                n2241 = Wait (ms)(milliseconds to wait=w3738) -> ()  [unwired: 1 out]
                                }
                                frame #10 {
                                n2242 = property on="Rescale on Mean" class="Bool (strict)"("Val(Sgnl)"=TRUE ("Value (Signaling)")) -> ()  [unwired: 2 in, 2 out]
                                }
                                }
                                }
                                frame "2", Default {
                                }
                              }
                            }
                          }
                        }
                      }
                      n2243 = Concatenate Strings("Formed tether in ", w3687, " attempt(s)." ("string")) -> (w3684:string)
                      n2244 = local read "Messages"() -> (w3691:string)
                      n2245 = local write "Fish for Tether"(w3693) -> ()
                      n2246 = call "Update messages.vi"("Message to add"=w3684, "Old message string"=w3691) -> ("New message string"=w3690:string)
                      n2247 = local write "Messages"(w3690) -> ()
                      n2248 = Get Date/Time In Seconds() -> (seconds since 1Jan1904=→"Time tether formed":timestamp)
                      "Tether" <- "Tether Alarm?"
                    }
                  }
                }
                frame #2 {
                  n2249 = local read "Oscillate Traps"() -> (w3743:bool)
                  n2250 = local read "Stop All"() -> (w3745:bool)
                  n2251 = Not Or(1:w3742, 2:w3743) -> (0:w3741:bool)
                  n2252 = Compound Arithmetic op=OR(w3745, w3741) -> (w3744:bool)
                }
              }
              n2253 = node-c288() -> ()  [unwired: 2 out]
            }
            n2254 = node-c288(w3601) -> ()  [unwired: 1 out]
          }
        }
      }
      event "Fl. Triggered...": Value Change {
        n2255 = event-data() -> ()  [unwired: 7 out]
        n2256 = case shown="True" "Fl. Triggered..." {
          frame False {
          }
          frame True {
            n2257 = node-c288() -> (w3757:T24)  [unwired: 4 out]
            n2258 = timed-loop {
              timing: w3757 -> [_]
              timing-out: [_] -> w3756
              tunnel: "Action" -> [w3761]
              shift-right: [w3758] -> _
              shift-left: u8 255 -> [w3760]
              stop <- w3762 stop-if-true
              n2259 = node-c288() -> ()  [unwired: 2 out]
              n2260 = flat-sequence {
                tunnel: w3761 -> [w3774]
                tunnel: w3760 -> [w3771]
                tunnel: [w3770] -> w3759
                tunnel: [w3860] -> w3762
                tunnel: w3759 -> [w3859]
                tunnel: [w3859] -> w3758
                frame #0 {
                  n2261 = local read "Delta Fl. 2"() -> (w3765:dbl)
                  n2262 = local read "Delta Fl. 1"() -> (w3766:dbl)
                  n2263 = Select(t=w3766, s="APD to Watch", f=w3765) -> (s? t:f=w3764:dbl)
                  n2264 = Multiply(x="Fl. Delta Thresh. (kHz)", y=1000.0) -> (x*y=w3773:dbl)
                  n2265 = Greater?(x=w3764, y=w3773) -> (0:w3768:bool)
                  n2266 = Or(x="Force Yank", y=w3768) -> (x .or. y?=w3769:bool)
                  n2267 = case shown="True" w3769 {
                    tunnel: w3774 -> [_ w3784]
                    tunnel: w3771 -> [w3776 w3780]
                    tunnel: [w3776 w3777] -> w3770
                    frame False {
                    }
                    frame True {
                      n2268 = flat-sequence {
                        tunnel: w3781 -> [w3790]
                        tunnel: [w3790] -> w3785
                        tunnel: w3784 -> [w3789]
                        tunnel: [w3789] -> w3783
                        tunnel: [w3788] -> w3782
                        tunnel: w3780 -> [w3787]
                        tunnel: [w3786] -> w3779
                        tunnel: w3785 -> [w3815]
                        tunnel: w3783 -> [w3814]
                        tunnel: w3782 -> [w3813]
                        tunnel: w3779 -> [w3812]
                        tunnel: [w3812] -> w3778
                        tunnel: w3778 -> [w3857]
                        tunnel: [w3857] -> w3777
                        frame #0 {
                          n2269 = call <vilib>:"Beep.vi"() -> ()  [unwired: 3 in, 9 out]
                          n2270 = local write "Waiting"(FALSE ("Waiting")) -> ()
                          n2271 = Increment(x=w3787) -> (x+1=w3786:u8)
                          n2272 = case shown="\"Yank\"" w3789 {
                            tunnel: w3786 -> [_ _ w3796]
                            frame "Image" {
                              n2273 = property on="Confocal Image" class="Bool (strict)"("Val(Sgnl)"=TRUE ("Value (Signaling)")) -> ()  [unwired: 2 in, 2 out]
                            }
                            frame "Alarm", Default {
                            }
                            frame "Yank" {
                              n2274 = flat-sequence {
                                tunnel: w3796 -> [w3799]
                                tunnel: [w3798] -> w3795
                                tunnel: ["N Array El"] -> w3794
                                tunnel: w3795 -> [w3809]
                                tunnel: w3794 -> [w3805]
                                frame #0 {
                                n2275 = Multiply(x="Yank Delay (s)", y=1000.0) -> (x*y=w3802:dbl)
                                n2276 = Quotient & Remainder(x=w3799, y="N Array El") -> (x-y*floor(x/y)=w3798:u8)  [unwired: 1 out]
                                n2277 = Wait (ms)(milliseconds to wait=w3802) -> ()  [unwired: 1 out]
                                }
                                frame #1 {
                                n2278 = Random Number (0-1)() -> (number: 0 to 1=w3806:dbl)
                                n2279 = Multiply(x=w3805, y=w3806) -> (x*y=w3804:dbl)
                                n2280 = Round Toward -Infinity(1:w3804) -> (0:w3803:dbl)
                                n2281 = Select(t=w3803, s="Random Choice", f=w3809) -> (s? t:f=w3807:dbl)
                                n2282 = Index Array(array="Yank to Delta Array (MHz)", index=w3807) -> (element=w3810:dbl)
                                n2283 = property on="Trap Delta (MHz)" class="DigNum (strict)"("Val(Sgnl)"=w3810) -> ()  [unwired: 2 in, 2 out]
                                }
                              }
                            }
                          }
                          n2284 = local read "Time (s)"() -> (w3788:dbl)
                          "Fl. High" <- TRUE ("Yanking")
                        }
                        frame #1 {
                          n2285 = node-c288() -> (w3817:T24)  [unwired: 4 out]
                          n2286 = timed-loop {
                            timing: w3817 -> [_]
                            timing-out: [_] -> w3816
                            tunnel: w3815 -> [w3833]
                            tunnel: w3814 -> [w3831]
                            tunnel: w3813 -> [w3830]
                            stop <- w3832 stop-if-true
                            n2287 = node-c288() -> ()  [unwired: 2 out]
                            n2288 = local read "Fl. Delta Thresh. (kHz)"() -> (w3825:dbl)
                            n2289 = local read "Fl. Triggered..."() -> (w3834:bool)
                            n2290 = local read "Delta Fl. 1"() -> (w3821:dbl)
                            n2291 = local read "Delta Fl. 2"() -> (w3819:dbl)
                            n2292 = local read "Stop All"() -> (w3828:bool)
                            n2293 = local read "APD to Watch"() -> (w3820:bool)
                            n2294 = Select(t=w3821, s=w3820, f=w3819) -> (s? t:f=w3818:dbl)
                            n2295 = Not(x=w3834) -> (.not. x?=w3829:bool)
                            n2296 = Multiply(x=w3825, y=1000.0) -> (x*y=w3824:dbl)
                            n2297 = Negate(x=w3824) -> (-x=w3823:dbl)
                            n2298 = Less?(x=w3818, y=w3823) -> (x < y?=w3827:bool)
                            n2299 = Compound Arithmetic op=OR(w3827, w3828, w3829, "Force Reset") -> (w3832:bool)
                            n2300 = case shown="True" w3832 {
                              tunnel: w3833 -> [_ w3845]
                              tunnel: w3831 -> [_ w3844]
                              tunnel: w3830 -> [_ w3842]
                              frame False {
                              }
                              frame True {
                                n2301 = case shown="\"Yank\"" w3844 {
                                tunnel: w3845 -> [_ w3846]
                                frame "Image", Default {
                                }
                                frame "Yank" {
                                n2302 = flat-sequence {
                                tunnel: [w3851] -> w3847
                                tunnel: w3846 -> [w3851]
                                tunnel: w3847 -> [w3852]
                                frame #0 {
                                n2303 = local read "Yank Delay (s)"() -> (w3850:dbl)
                                n2304 = Multiply(x=w3850, y=1000.0) -> (x*y=w3848:dbl)
                                n2305 = Wait (ms)(milliseconds to wait=w3848) -> ()  [unwired: 1 out]
                                }
                                frame #1 {
                                n2306 = property on="Trap Delta (MHz)" class="DigNum (strict)"("Val(Sgnl)"=w3852) -> ()  [unwired: 2 in, 2 out]
                                }
                                }
                                }
                                }
                                n2307 = local read "Time (s)"() -> (w3843:dbl)
                                n2308 = Subtract(x=w3843, y=w3842) -> (x-y=w3839:dbl)
                                "Duration (s)" <- w3839
                                n2309 = Number To Decimal String(number=w3839, width (-)=i16 0) -> (decimal integer string=w3837:string)
                                n2310 = Concatenate Strings(w3837, " s fluorescence event." ("string")) -> (w3835:string)
                                n2311 = local read "Messages"() -> (w3841:string)
                                n2312 = call "Update messages.vi"("Message to add"=w3835, "Old message string"=w3841) -> ("New message string"=w3840:string)
                                n2313 = call <vilib>:"Beep.vi"() -> ()  [unwired: 3 in, 9 out]
                                n2314 = local write "Messages"(w3840) -> ()
                              }
                            }
                            n2315 = node-c288() -> ()  [unwired: 2 out]
                          }
                          n2316 = node-c288(w3816) -> ()  [unwired: 1 out]
                        }
                        frame #2 {
                          n2317 = local write "Fl. High"(FALSE ("Yanking")) -> ()
                        }
                      }
                      n2318 = local read "Trap Delta (MHz)"() -> (w3781:dbl)
                    }
                  }
                }
                frame #1 {
                  n2319 = local read "Stop All"() -> (w3863:bool)
                  n2320 = local read "Fl. Triggered..."() -> (w3861:bool)
                  n2321 = Not(x=w3861) -> (.not. x?=w3862:bool)
                  n2322 = Or(x=w3862, y=w3863) -> (x .or. y?=w3860:bool)
                  n2323 = Not(x=w3860) -> (.not. x?=→"Waiting":bool)
                }
              }
              n2324 = node-c288() -> ()  [unwired: 2 out]
            }
            n2325 = node-c288(w3756) -> ()  [unwired: 1 out]
          }
        }
      }
      event "Stop All": Value Change {
        n2326 = event-data() -> ()  [unwired: 7 out]
        n2327 = local read "Stop All"() -> (w3869:bool)
      }
    }
    n2328 = node-c288() -> ()  [unwired: 2 out]
  }
  n2329 = node-c288(w76) -> ()  [unwired: 1 out]
  n2330 = node-c288(w165) -> ()  [unwired: 1 out]
  n2331 = flat-sequence {
    tunnel: w37 -> [w3874]
    tunnel: [w3873] -> w43
    tunnel: [w3870] -> w42
    tunnel: w41 -> [_]
    tunnel: w40 -> [_]
    tunnel: w39 -> [_]
    tunnel: w38 -> [_]
    tunnel: w36 -> [w3871]
    tunnel: w43 -> [w3877]
    tunnel: w42 -> [w3876]
    frame #0 {
      w3872 = FALSE ("APD to FIFO")
      n2332 = xnode "Read/Write Control"("FPGA VI Reference In"=w3874, "error in"=w3871, "APD to FIFO"=w3872, "AI to FIFO"=w3872) -> ("FPGA VI Reference Out"=w3873:T19, "error out"=w3870:errorcluster)
    }
    frame #1 {
      n2333 = xnode "Invoke Method"("FPGA VI Reference In"=w3877, "error in"=w3876) -> ("FPGA VI Reference Out"=w3875:T19)  [unwired: 1 out]
      n2334 = xnode "Close FPGA VI Reference"("FPGA VI Reference In"=w3875) -> ()  [unwired: 1 in, 1 out]
    }
  }
